vi "ToEng_poly.VI"   [LabVIEW 2019, in "DAQ_Engine.lvclass"]
doc: "Developed by Kevin Thompson\nkevin@thompsonengineering.net\n\nCopyright 2020\nThompson Engineering, LLC\nConverts raw A/D measurements from binary counts to engineering units (volts or mAmps, for example)."
uses:
  DAQ_Engine.lvclass
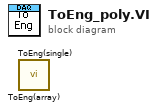
[diagram p0: block diagram]
diagram:
  n1 = call "ToEng(array).vi"() -> ()  [unwired: 3 in, 2 out]
  n2 = call "ToEng(single).VI"() -> ()  [unwired: 3 in, 2 out]
